vi "HandleObservationSync.vi"(8 "error in (no error)":errorcluster, 11 "S4GUI in":refnum<class "S4GUI.lvclass">) -> (0 "error out":errorcluster, 3 "S4GUI out":refnum<class "S4GUI.lvclass">)   [LabVIEW 2018, in "S4GUI.lvclass"] (continued)
              n490 = Build Array(w1193, w1192, w1191, w1190) -> (w1195:bool[])
              n491 = Boolean Array To Number(Boolean array=w1195) -> (number=w1194:u32)
              n492 = Number To Decimal String(number=w1194) -> (decimal integer string=w1188:string)  [unwired: 1 in]
              n493 = Concatenate Strings("CHANNEL ERROR < " ("string"), w1188, ">: Initialization failed. S4GUI:HandleObservationSync.vi state 252." ("Error Msg")) -> (w1187:string)
              n494 = Bundle By Name(cluster=w1198, "Obs_state"=u32 1, "Error Msg"=w1187) -> (w1197:refnum<class "S4GUI.lvclass">)
            }
            frame 2 {
              n495 = Build Array(w1208, w1207, w1206, w1205) -> (w1204:bool[])
              n496 = Boolean Array To Number(Boolean array=w1204) -> (number=w1200:u32)
              n497 = Number To Decimal String(number=w1200) -> (decimal integer string=w1199:string)  [unwired: 1 in]
              n498 = Concatenate Strings("CHANNEL ERROR < " ("string"), w1199, ">:  Invalid Exposition Time. S4GUI:HandleObservationSync.vi state 252." ("Error Msg")) -> (w1202:string)
              n499 = Bundle By Name(cluster=w1211, "Obs_state"=u32 1, "Error Msg"=w1202) -> (w1210:refnum<class "S4GUI.lvclass">)
            }
            frame 3 {
              n500 = Bundle By Name(cluster=w1215, "Obs_state"=u32 1, "Error Msg"="ERROR: Invalid configuration in the channels. S4GUI:HandleObservationSync.vi state 252.") -> (w1214:refnum<class "S4GUI.lvclass">)
            }
          }
        }
        frame 253 {
          # "Sem SyncBox, \ntrigger mode = 0 (internal)\nCom SyncBox\ntrigger mode = 6 (ext. start)"
          n501 = call-dynamic "Read Sync Box.lvclass.vi"("error in (no error)"=w1327, "SPARC4_AC in"=w1326) -> ("error out"=w1329:errorcluster, "Sync Box.lvclass"=w1330:refnum<class "Sync Box.lvclass">, "SPARC4_AC out"=w1325:refnum<class "S4GUI.lvclass">)  [unwired: 7 in]
          n502 = call "Read connection.vi"("error in (no error)"=w1329, "Server in"=w1330) -> ("error out"=w1328:errorcluster, "connection"=w1290:bool)  [unwired: 7 in, 1 out]
          n503 = case shown="True" w1290 {
            tunnel: [u8 6 ("TRIGGER_MODE") u8 0 ("TRIGGER_MODE")] -> w1307
            frame True {
            }
            frame False {
            }
          }
          n504 = call-dynamic "Read AcquisitionA.vi"("error in (no error)"=w1328, "S4ACS_GUI in"=w1325) -> ("error out"=w1312:errorcluster, "Acquisition.lvclass"=w1313:refnum<class "Acquisition.lvclass">, "S4ACS_GUI out"=w1311:refnum<class "S4GUI.lvclass">)  [unwired: 7 in]
          n505 = call-dynamic "Read Channel.vi"("error in (no error)"=w1312, "Acquisition in"=w1313) -> ("error out"=w1295:errorcluster, "Channel.lvclass"=w1294:refnum<class "Channel.lvclass">, "Acquisition out"=w1322:refnum<class "Acquisition.lvclass">)  [unwired: 7 in]
          n506 = call-dynamic "Read Interface.vi"("error in (no error)"=w1295, "Channel in"=w1294) -> ("error out"=w1293:errorcluster, "Interface.lvclass"=w1299:refnum<class "Interface.lvclass">, "Channel out"=w1298:refnum<class "Channel.lvclass">)  [unwired: 7 in]
          n507 = call-dynamic "Get CCD_Config.vi"("error in (no error)"=w1293, "Interface in"=w1299) -> ("error out"=w1306:errorcluster, "output cluster"=w1308:T1, "Interface out"=w1305:refnum<class "Interface.lvclass">)  [unwired: 7 in]
          n508 = Bundle By Name(cluster=w1308, "TRIGGER_MODE"=w1307) -> (w1304:T1)
          n509 = call-dynamic "Set CCD_Config.vi"("error in (no error)"=w1306, "input cluster"=w1304, "Interface in"=w1305) -> ("error out"=w1302:errorcluster, "Interface out"=w1300:refnum<class "Interface.lvclass">)  [unwired: 7 in]
          n510 = Flatten To String(anything=w1304, error in (no error)=w1302) -> (data string=w1303:string, error out=w1301:errorcluster)  [unwired: 2 in, 1 out]
          n511 = call "Write flatted cluster.vi"("error in (no error)"=w1301, "flatted cluster"=w1303, "Interface in"=w1300) -> ("error out"=w1296:errorcluster, "Interface out"=w1297:refnum<class "Interface.lvclass">)  [unwired: 7 in]
          n512 = Increment(x=w1333) -> (x+1=w1332:u32)
          n513 = call-dynamic "Write Interface.vi"("error in (no error)"=w1296, "Interface.lvclass"=w1297, "Channel in"=w1298) -> ("error out"=w1292:errorcluster, "Channel out"=w1291:refnum<class "Channel.lvclass">)  [unwired: 7 in]
          n514 = call-dynamic "Read State Machine.vi"("error in (no error)"=w1292, "Device in"=w1291) -> ("error out"=w1319:errorcluster, "State Machine.lvclass"=w1321:refnum<class "State Machine.lvclass">, "Device out"=w1317:refnum<class "Channel.lvclass">)  [unwired: 7 in]
          n515 = call "Next State.vi"("error in (no error)"=w1319, "New_State"=60, "State Machine in"=w1321) -> ("error out"=w1314:errorcluster, "State Machine out"=w1315:refnum<class "State Machine.lvclass">)  [unwired: 7 in]
          n516 = call-dynamic "Write State Machine.vi"("error in (no error)"=w1314, "State Machine.lvclass"=w1315, "Device in"=w1317) -> ("error out"=w1316:errorcluster, "Device out"=w1318:refnum<class "Channel.lvclass">)  [unwired: 7 in]
          n517 = call-dynamic "Write Channel.vi"("error in (no error)"=w1316, "Channel.lvclass"=w1318, "Acquisition in"=w1322) -> ("error out"=w1309:errorcluster, "Acquisition out"=w1310:refnum<class "Acquisition.lvclass">)  [unwired: 7 in]
          n518 = call-dynamic "Write AcquisitionA.vi"("error in (no error)"=w1309, "Acquisition.lvclass"=w1310, "S4ACS_GUI in"=w1311) -> ("error out"=w1324:errorcluster, "S4ACS_GUI out"=w1323:refnum<class "S4GUI.lvclass">)  [unwired: 7 in]
          n519 = Bundle By Name(cluster=w1323, "Obs_state"=w1332) -> (w1331:refnum<class "S4GUI.lvclass">)
        }
        frame 254 {
          # "Espera terminar a execução do comando atual \nantes de ir ao proximo passo da Observação."
          n520 = call-dynamic "Read AcquisitionA.vi"("error in (no error)"=w1353, "S4ACS_GUI in"=w1354) -> ("error out"=w1359:errorcluster, "Acquisition.lvclass"=w1360:refnum<class "Acquisition.lvclass">, "S4ACS_GUI out"=w1356:refnum<class "S4GUI.lvclass">)  [unwired: 7 in]
          n521 = call-dynamic "Read Channel.vi"("error in (no error)"=w1359, "Acquisition in"=w1360) -> ("error out"=w1351:errorcluster, "Channel.lvclass"=w1350:refnum<class "Channel.lvclass">, "Acquisition out"=w1358:refnum<class "Acquisition.lvclass">)  [unwired: 7 in]
          n522 = call-dynamic "Read State Machine.vi"("error in (no error)"=w1351, "Device in"=w1350) -> ("error out"=w1342:errorcluster, "State Machine.lvclass"=w1344:refnum<class "State Machine.lvclass">, "Device out"=w1348:refnum<class "Channel.lvclass">)  [unwired: 7 in]
          n523 = call-dynamic "Read State.vi"("error in (no error)"=w1342, "State Machine in"=w1344) -> ("error out"=w1341:errorcluster, "State"=w1338:i32, "State Machine out"=w1343:refnum<class "State Machine.lvclass">)  [unwired: 7 in]
          n524 = Equal To 0?(x=w1338) -> (x = 0?=w1340:bool)
          n525 = call-dynamic "Write State Machine.vi"("error in (no error)"=w1341, "State Machine.lvclass"=w1343, "Device in"=w1348) -> ("error out"=w1347:errorcluster, "Device out"=w1349:refnum<class "Channel.lvclass">)  [unwired: 7 in]
          n526 = call-dynamic "Write Channel.vi"("error in (no error)"=w1347, "Channel.lvclass"=w1349, "Acquisition in"=w1358) -> ("error out"=w1355:errorcluster, "Acquisition out"=w1357:refnum<class "Acquisition.lvclass">)  [unwired: 7 in]
          n527 = disable-structure shown="Enabled" {
            disable-tunnel: [u32 299 ("t") w1362] -> w1337
            disable-tunnel: w1336 -> [_ w1363]
            frame Disabled {
            }
            frame Enabled {
              n528 = Increment(x=w1363) -> (x+1=w1362:u32)
            }
          }
          n529 = Select(t=w1337, s=w1340, f=w1336) -> (s? t:f=w1339:u32)
          n530 = call-dynamic "Write AcquisitionA.vi"("error in (no error)"=w1355, "Acquisition.lvclass"=w1357, "S4ACS_GUI in"=w1356) -> ("error out"=w1352:errorcluster, "S4ACS_GUI out"=w1346:refnum<class "S4GUI.lvclass">)  [unwired: 7 in]
          n531 = Bundle By Name(cluster=w1346, "Obs_state"=w1339) -> (w1345:refnum<class "S4GUI.lvclass">)
        }
        frame 255 {
          n532 = call "Read AcquisitionB.vi"("error in (no error)"=w1374, "S4ACS_GUI in"=w1375) -> ("error out"=w1367:errorcluster, "Acquisition.lvclass"=w1368:refnum<class "Acquisition.lvclass">, "S4ACS_GUI out"=w1377:refnum<class "S4GUI.lvclass">)  [unwired: 7 in]
          n533 = call "Read connection.vi"("error in (no error)"=w1367, "Server in"=w1368) -> ("error out"=w1366:errorcluster, "connection"=w1364:bool, "Server out"=w1365:refnum<class "Acquisition.lvclass">)  [unwired: 7 in]
          n534 = case shown="False" w1364 {
            tunnel: w1365 -> [w1385 w1405]
            tunnel: w1366 -> [w1384 w1404]
            tunnel: [w1385 w1402] -> w1378
            tunnel: [w1384 w1401] -> w1376
            tunnel: w1371 -> [w1383 w1394]
            tunnel: [w1379 w1393] -> w1370
            frame False {
              n535 = Increment(x=w1383) -> (x+1=w1382:u32)
              n536 = Increment(x=w1382) -> (x+1=w1381:u32)
              n537 = Increment(x=w1381) -> (x+1=w1380:u32)
              n538 = Increment(x=w1380) -> (x+1=w1379:u32)
            }
            frame True {
              # "configura o canal,\nmas não dispara\na exposicao."
              n539 = call-dynamic "Read Channel.vi"("error in (no error)"=w1404, "Acquisition in"=w1405) -> ("error out"=w1390:errorcluster, "Channel.lvclass"=w1392:refnum<class "Channel.lvclass">, "Acquisition out"=w1403:refnum<class "Acquisition.lvclass">)  [unwired: 7 in]
              n540 = call-dynamic "Write expose.vi"("error in (no error)"=w1390, "expose"=FALSE, "Channel in"=w1392) -> ("error out"=w1389:errorcluster, "Channel out"=w1391:refnum<class "Channel.lvclass">)  [unwired: 7 in]
              n541 = call-dynamic "Read State Machine.vi"("error in (no error)"=w1389, "Device in"=w1391) -> ("error out"=w1398:errorcluster, "State Machine.lvclass"=w1400:refnum<class "State Machine.lvclass">, "Device out"=w1396:refnum<class "Channel.lvclass">)  [unwired: 7 in]
              n542 = call "Next State.vi"("error in (no error)"=w1398, "New_State"=1, "State Machine in"=w1400) -> ("error out"=w1386:errorcluster, "State Machine out"=w1387:refnum<class "State Machine.lvclass">)  [unwired: 7 in]
              n543 = Increment(x=w1394) -> (x+1=w1393:u32)
              n544 = call-dynamic "Write State Machine.vi"("error in (no error)"=w1386, "State Machine.lvclass"=w1387, "Device in"=w1396) -> ("error out"=w1395:errorcluster, "Device out"=w1397:refnum<class "Channel.lvclass">)  [unwired: 7 in]
              n545 = call-dynamic "Write Channel.vi"("error in (no error)"=w1395, "Channel.lvclass"=w1397, "Acquisition in"=w1403) -> ("error out"=w1401:errorcluster, "Acquisition out"=w1402:refnum<class "Acquisition.lvclass">)  [unwired: 7 in]
            }
          }
          n546 = call "Write AcquisitionB.vi"("error in (no error)"=w1376, "Acquisition.lvclass"=w1378, "S4ACS_GUI in"=w1377) -> ("error out"=w1373:errorcluster, "S4ACS_GUI out"=w1372:refnum<class "S4GUI.lvclass">)  [unwired: 7 in]
          n547 = Bundle By Name(cluster=w1372, "Obs_state"=w1370) -> (w1369:refnum<class "S4GUI.lvclass">)
        }
        frame 256 {
          # "Espera terminar a execução do comando atual \nantes de ir ao proximo passo da Observação."
          n548 = call "Read AcquisitionB.vi"("error in (no error)"=w1423, "S4ACS_GUI in"=w1424) -> ("error out"=w1429:errorcluster, "Acquisition.lvclass"=w1430:refnum<class "Acquisition.lvclass">, "S4ACS_GUI out"=w1426:refnum<class "S4GUI.lvclass">)  [unwired: 7 in]
          n549 = call-dynamic "Read Channel.vi"("error in (no error)"=w1429, "Acquisition in"=w1430) -> ("error out"=w1421:errorcluster, "Channel.lvclass"=w1420:refnum<class "Channel.lvclass">, "Acquisition out"=w1428:refnum<class "Acquisition.lvclass">)  [unwired: 7 in]
          n550 = call-dynamic "Read State Machine.vi"("error in (no error)"=w1421, "Device in"=w1420) -> ("error out"=w1412:errorcluster, "State Machine.lvclass"=w1414:refnum<class "State Machine.lvclass">, "Device out"=w1418:refnum<class "Channel.lvclass">)  [unwired: 7 in]
          n551 = call-dynamic "Read State.vi"("error in (no error)"=w1412, "State Machine in"=w1414) -> ("error out"=w1411:errorcluster, "State"=w1408:i32, "State Machine out"=w1413:refnum<class "State Machine.lvclass">)  [unwired: 7 in]
          n552 = call-dynamic "Write State Machine.vi"("error in (no error)"=w1411, "State Machine.lvclass"=w1413, "Device in"=w1418) -> ("error out"=w1417:errorcluster, "Device out"=w1419:refnum<class "Channel.lvclass">)  [unwired: 7 in]
          n553 = call-dynamic "Write Channel.vi"("error in (no error)"=w1417, "Channel.lvclass"=w1419, "Acquisition in"=w1428) -> ("error out"=w1425:errorcluster, "Acquisition out"=w1427:refnum<class "Acquisition.lvclass">)  [unwired: 7 in]
          n554 = Equal To 0?(x=w1408) -> (x = 0?=w1410:bool)
          n555 = disable-structure shown="Enabled" {
            disable-tunnel: [u32 299 ("t") w1432] -> w1406
            disable-tunnel: w1407 -> [_ w1435]
            frame Disabled {
            }
            frame Enabled {
              n556 = Increment(x=w1435) -> (x+1=w1434:u32)
              n557 = Increment(x=w1434) -> (x+1=w1433:u32)
              n558 = Increment(x=w1433) -> (x+1=w1432:u32)
            }
          }
          n559 = Select(t=w1406, s=w1410, f=w1407) -> (s? t:f=w1409:u32)
          n560 = call "Write AcquisitionB.vi"("error in (no error)"=w1425, "Acquisition.lvclass"=w1427, "S4ACS_GUI in"=w1426) -> ("error out"=w1422:errorcluster, "S4ACS_GUI out"=w1416:refnum<class "S4GUI.lvclass">)  [unwired: 7 in]
          n561 = Bundle By Name(cluster=w1416, "Obs_state"=w1409) -> (w1415:refnum<class "S4GUI.lvclass">)
        }
        frame 257 {
          # "Sem SyncBox, \ntrigger mode = 0 (internal)\nCom SyncBox\ntrigger mode = 6 (ext. start)"
          n562 = call-dynamic "Read Sync Box.lvclass.vi"("error in (no error)"=w1473, "SPARC4_AC in"=w1472) -> ("error out"=w1475:errorcluster, "Sync Box.lvclass"=w1476:refnum<class "Sync Box.lvclass">, "SPARC4_AC out"=w1471:refnum<class "S4GUI.lvclass">)  [unwired: 7 in]
          n563 = call "Read connection.vi"("error in (no error)"=w1475, "Server in"=w1476) -> ("error out"=w1474:errorcluster, "connection"=w1437:bool)  [unwired: 7 in, 1 out]
          n564 = case shown="False" w1437 {
            tunnel: [u8 6 ("TRIGGER_MODE") u8 0 ("TRIGGER_MODE")] -> w1436
            frame True {
            }
            frame False {
            }
          }
          n565 = call "Read AcquisitionB.vi"("error in (no error)"=w1474, "S4ACS_GUI in"=w1471) -> ("error out"=w1458:errorcluster, "Acquisition.lvclass"=w1459:refnum<class "Acquisition.lvclass">, "S4ACS_GUI out"=w1457:refnum<class "S4GUI.lvclass">)  [unwired: 7 in]
          n566 = call-dynamic "Read Channel.vi"("error in (no error)"=w1458, "Acquisition in"=w1459) -> ("error out"=w1442:errorcluster, "Channel.lvclass"=w1441:refnum<class "Channel.lvclass">, "Acquisition out"=w1468:refnum<class "Acquisition.lvclass">)  [unwired: 7 in]
          n567 = call-dynamic "Read Interface.vi"("error in (no error)"=w1442, "Channel in"=w1441) -> ("error out"=w1440:errorcluster, "Interface.lvclass"=w1446:refnum<class "Interface.lvclass">, "Channel out"=w1445:refnum<class "Channel.lvclass">)  [unwired: 7 in]
          n568 = call-dynamic "Get CCD_Config.vi"("error in (no error)"=w1440, "Interface in"=w1446) -> ("error out"=w1453:errorcluster, "output cluster"=w1454:T1, "Interface out"=w1452:refnum<class "Interface.lvclass">)  [unwired: 7 in]
          n569 = Bundle By Name(cluster=w1454, "TRIGGER_MODE"=w1436) -> (w1451:T1)
          n570 = call-dynamic "Set CCD_Config.vi"("error in (no error)"=w1453, "input cluster"=w1451, "Interface in"=w1452) -> ("error out"=w1449:errorcluster, "Interface out"=w1447:refnum<class "Interface.lvclass">)  [unwired: 7 in]
          n571 = Flatten To String(anything=w1451, error in (no error)=w1449) -> (data string=w1450:string, error out=w1448:errorcluster)  [unwired: 2 in, 1 out]
          n572 = call "Write flatted cluster.vi"("error in (no error)"=w1448, "flatted cluster"=w1450, "Interface in"=w1447) -> ("error out"=w1443:errorcluster, "Interface out"=w1444:refnum<class "Interface.lvclass">)  [unwired: 7 in]
          n573 = Increment(x=w1479) -> (x+1=w1478:u32)
          n574 = call-dynamic "Write Interface.vi"("error in (no error)"=w1443, "Interface.lvclass"=w1444, "Channel in"=w1445) -> ("error out"=w1439:errorcluster, "Channel out"=w1438:refnum<class "Channel.lvclass">)  [unwired: 7 in]
          n575 = call-dynamic "Read State Machine.vi"("error in (no error)"=w1439, "Device in"=w1438) -> ("error out"=w1465:errorcluster, "State Machine.lvclass"=w1467:refnum<class "State Machine.lvclass">, "Device out"=w1463:refnum<class "Channel.lvclass">)  [unwired: 7 in]
          n576 = call "Next State.vi"("error in (no error)"=w1465, "New_State"=60, "State Machine in"=w1467) -> ("error out"=w1460:errorcluster, "State Machine out"=w1461:refnum<class "State Machine.lvclass">)  [unwired: 7 in]
          n577 = call-dynamic "Write State Machine.vi"("error in (no error)"=w1460, "State Machine.lvclass"=w1461, "Device in"=w1463) -> ("error out"=w1462:errorcluster, "Device out"=w1464:refnum<class "Channel.lvclass">)  [unwired: 7 in]
          n578 = call-dynamic "Write Channel.vi"("error in (no error)"=w1462, "Channel.lvclass"=w1464, "Acquisition in"=w1468) -> ("error out"=w1455:errorcluster, "Acquisition out"=w1456:refnum<class "Acquisition.lvclass">)  [unwired: 7 in]
          n579 = call "Write AcquisitionB.vi"("error in (no error)"=w1455, "Acquisition.lvclass"=w1456, "S4ACS_GUI in"=w1457) -> ("error out"=w1470:errorcluster, "S4ACS_GUI out"=w1469:refnum<class "S4GUI.lvclass">)  [unwired: 7 in]
          n580 = Bundle By Name(cluster=w1469, "Obs_state"=w1478) -> (w1477:refnum<class "S4GUI.lvclass">)
        }
        frame 258 {
          # "Espera terminar a execução do comando atual \nantes de ir ao proximo passo da Observação."
          n581 = call "Read AcquisitionB.vi"("error in (no error)"=w1499, "S4ACS_GUI in"=w1500) -> ("error out"=w1505:errorcluster, "Acquisition.lvclass"=w1506:refnum<class "Acquisition.lvclass">, "S4ACS_GUI out"=w1502:refnum<class "S4GUI.lvclass">)  [unwired: 7 in]
          n582 = call-dynamic "Read Channel.vi"("error in (no error)"=w1505, "Acquisition in"=w1506) -> ("error out"=w1497:errorcluster, "Channel.lvclass"=w1496:refnum<class "Channel.lvclass">, "Acquisition out"=w1504:refnum<class "Acquisition.lvclass">)  [unwired: 7 in]
          n583 = call-dynamic "Read State Machine.vi"("error in (no error)"=w1497, "Device in"=w1496) -> ("error out"=w1488:errorcluster, "State Machine.lvclass"=w1490:refnum<class "State Machine.lvclass">, "Device out"=w1494:refnum<class "Channel.lvclass">)  [unwired: 7 in]
          n584 = call-dynamic "Read State.vi"("error in (no error)"=w1488, "State Machine in"=w1490) -> ("error out"=w1487:errorcluster, "State"=w1484:i32, "State Machine out"=w1489:refnum<class "State Machine.lvclass">)  [unwired: 7 in]
          n585 = call-dynamic "Write State Machine.vi"("error in (no error)"=w1487, "State Machine.lvclass"=w1489, "Device in"=w1494) -> ("error out"=w1493:errorcluster, "Device out"=w1495:refnum<class "Channel.lvclass">)  [unwired: 7 in]
          n586 = call-dynamic "Write Channel.vi"("error in (no error)"=w1493, "Channel.lvclass"=w1495, "Acquisition in"=w1504) -> ("error out"=w1501:errorcluster, "Acquisition out"=w1503:refnum<class "Acquisition.lvclass">)  [unwired: 7 in]
          n587 = Equal To 0?(x=w1484) -> (x = 0?=w1486:bool)
          n588 = Increment(x=w1483) -> (x+1=w1482:u32)
          n589 = Select(t=w1482, s=w1486, f=w1483) -> (s? t:f=w1485:u32)
          n590 = call "Write AcquisitionB.vi"("error in (no error)"=w1501, "Acquisition.lvclass"=w1503, "S4ACS_GUI in"=w1502) -> ("error out"=w1498:errorcluster, "S4ACS_GUI out"=w1492:refnum<class "S4GUI.lvclass">)  [unwired: 7 in]
          n591 = Bundle By Name(cluster=w1492, "Obs_state"=w1485) -> (w1491:refnum<class "S4GUI.lvclass">)
        }
        frame 259 {
          n592 = call-dynamic "Read AcquisitionC.vi"("error in (no error)"=w1517, "S4ACS_GUI in"=w1518) -> ("error out"=w1509:errorcluster, "Acquisition.lvclass"=w1511:refnum<class "Acquisition.lvclass">, "S4ACS_GUI out"=w1520:refnum<class "S4GUI.lvclass">)  [unwired: 7 in]
          n593 = call "Read connection.vi"("error in (no error)"=w1509, "Server in"=w1511) -> ("error out"=w1508:errorcluster, "connection"=w1507:bool, "Server out"=w1510:refnum<class "Acquisition.lvclass">)  [unwired: 7 in]
          n594 = case shown="True" w1507 {
            tunnel: w1510 -> [w1527 w1548]
            tunnel: w1508 -> [w1528 w1547]
            tunnel: [w1527 w1545] -> w1521
            tunnel: [w1528 w1544] -> w1519
            tunnel: w1514 -> [w1526 w1537]
            tunnel: [w1522 w1536] -> w1513
            frame False {
              n595 = Increment(x=w1526) -> (x+1=w1525:u32)
              n596 = Increment(x=w1525) -> (x+1=w1524:u32)
              n597 = Increment(x=w1524) -> (x+1=w1523:u32)
              n598 = Increment(x=w1523) -> (x+1=w1522:u32)
            }
            frame True {
              # "configura o canal,\nmas não dispara\na exposicao."
              n599 = call-dynamic "Read Channel.vi"("error in (no error)"=w1547, "Acquisition in"=w1548) -> ("error out"=w1533:errorcluster, "Channel.lvclass"=w1535:refnum<class "Channel.lvclass">, "Acquisition out"=w1546:refnum<class "Acquisition.lvclass">)  [unwired: 7 in]
              n600 = call-dynamic "Write expose.vi"("error in (no error)"=w1533, "expose"=FALSE, "Channel in"=w1535) -> ("error out"=w1532:errorcluster, "Channel out"=w1534:refnum<class "Channel.lvclass">)  [unwired: 7 in]
              n601 = call-dynamic "Read State Machine.vi"("error in (no error)"=w1532, "Device in"=w1534) -> ("error out"=w1541:errorcluster, "State Machine.lvclass"=w1543:refnum<class "State Machine.lvclass">, "Device out"=w1539:refnum<class "Channel.lvclass">)  [unwired: 7 in]
              n602 = call "Next State.vi"("error in (no error)"=w1541, "New_State"=1, "State Machine in"=w1543) -> ("error out"=w1529:errorcluster, "State Machine out"=w1530:refnum<class "State Machine.lvclass">)  [unwired: 7 in]
              n603 = Increment(x=w1537) -> (x+1=w1536:u32)
              n604 = call-dynamic "Write State Machine.vi"("error in (no error)"=w1529, "State Machine.lvclass"=w1530, "Device in"=w1539) -> ("error out"=w1538:errorcluster, "Device out"=w1540:refnum<class "Channel.lvclass">)  [unwired: 7 in]
              n605 = call-dynamic "Write Channel.vi"("error in (no error)"=w1538, "Channel.lvclass"=w1540, "Acquisition in"=w1546) -> ("error out"=w1544:errorcluster, "Acquisition out"=w1545:refnum<class "Acquisition.lvclass">)  [unwired: 7 in]
            }
          }
          n606 = call-dynamic "Write AcquisitionC.vi"("error in (no error)"=w1519, "Acquisition.lvclass"=w1521, "S4ACS_GUI in"=w1520) -> ("error out"=w1516:errorcluster, "S4ACS_GUI out"=w1515:refnum<class "S4GUI.lvclass">)  [unwired: 7 in]
          n607 = Bundle By Name(cluster=w1515, "Obs_state"=w1513) -> (w1512:refnum<class "S4GUI.lvclass">)
        }
        frame 260 {
          # "Espera terminar a execução do comando atual \nantes de ir ao proximo passo da Observação."
          n608 = call-dynamic "Read AcquisitionC.vi"("error in (no error)"=w1566, "S4ACS_GUI in"=w1567) -> ("error out"=w1572:errorcluster, "Acquisition.lvclass"=w1573:refnum<class "Acquisition.lvclass">, "S4ACS_GUI out"=w1569:refnum<class "S4GUI.lvclass">)  [unwired: 7 in]
          n609 = call-dynamic "Read Channel.vi"("error in (no error)"=w1572, "Acquisition in"=w1573) -> ("error out"=w1564:errorcluster, "Channel.lvclass"=w1563:refnum<class "Channel.lvclass">, "Acquisition out"=w1571:refnum<class "Acquisition.lvclass">)  [unwired: 7 in]
          n610 = call-dynamic "Read State Machine.vi"("error in (no error)"=w1564, "Device in"=w1563) -> ("error out"=w1555:errorcluster, "State Machine.lvclass"=w1557:refnum<class "State Machine.lvclass">, "Device out"=w1561:refnum<class "Channel.lvclass">)  [unwired: 7 in]
          n611 = call-dynamic "Read State.vi"("error in (no error)"=w1555, "State Machine in"=w1557) -> ("error out"=w1554:errorcluster, "State"=w1551:i32, "State Machine out"=w1556:refnum<class "State Machine.lvclass">)  [unwired: 7 in]
          n612 = Equal To 0?(x=w1551) -> (x = 0?=w1553:bool)
          n613 = call-dynamic "Write State Machine.vi"("error in (no error)"=w1554, "State Machine.lvclass"=w1556, "Device in"=w1561) -> ("error out"=w1560:errorcluster, "Device out"=w1562:refnum<class "Channel.lvclass">)  [unwired: 7 in]
          n614 = call-dynamic "Write Channel.vi"("error in (no error)"=w1560, "Channel.lvclass"=w1562, "Acquisition in"=w1571) -> ("error out"=w1568:errorcluster, "Acquisition out"=w1570:refnum<class "Acquisition.lvclass">)  [unwired: 7 in]
          n615 = disable-structure shown="Enabled" {
            disable-tunnel: [u32 299 ("t") w1575] -> w1549
            disable-tunnel: w1550 -> [_ w1578]
            frame Disabled {
            }
            frame Enabled {
              n616 = Increment(x=w1578) -> (x+1=w1577:u32)
              n617 = Increment(x=w1577) -> (x+1=w1576:u32)
              n618 = Increment(x=w1576) -> (x+1=w1575:u32)
            }
          }
          n619 = Select(t=w1549, s=w1553, f=w1550) -> (s? t:f=w1552:u32)
          n620 = call-dynamic "Write AcquisitionC.vi"("error in (no error)"=w1568, "Acquisition.lvclass"=w1570, "S4ACS_GUI in"=w1569) -> ("error out"=w1565:errorcluster, "S4ACS_GUI out"=w1559:refnum<class "S4GUI.lvclass">)  [unwired: 7 in]
          n621 = Bundle By Name(cluster=w1559, "Obs_state"=w1552) -> (w1558:refnum<class "S4GUI.lvclass">)
        }
        frame 261 {
          # "Sem SyncBox, \ntrigger mode = 0 (internal)\nCom SyncBox\ntrigger mode = 6 (ext. start)"
          n622 = call-dynamic "Read Sync Box.lvclass.vi"("error in (no error)"=w1616, "SPARC4_AC in"=w1615) -> ("error out"=w1618:errorcluster, "Sync Box.lvclass"=w1619:refnum<class "Sync Box.lvclass">, "SPARC4_AC out"=w1614:refnum<class "S4GUI.lvclass">)  [unwired: 7 in]
          n623 = call "Read connection.vi"("error in (no error)"=w1618, "Server in"=w1619) -> ("error out"=w1617:errorcluster, "connection"=w1580:bool)  [unwired: 7 in, 1 out]
          n624 = case shown="False" w1580 {
            tunnel: [u8 6 ("TRIGGER_MODE") u8 0 ("TRIGGER_MODE")] -> w1579
            frame True {
            }
            frame False {
            }
          }
          n625 = call-dynamic "Read AcquisitionC.vi"("error in (no error)"=w1617, "S4ACS_GUI in"=w1614) -> ("error out"=w1601:errorcluster, "Acquisition.lvclass"=w1602:refnum<class "Acquisition.lvclass">, "S4ACS_GUI out"=w1600:refnum<class "S4GUI.lvclass">)  [unwired: 7 in]
          n626 = call-dynamic "Read Channel.vi"("error in (no error)"=w1601, "Acquisition in"=w1602) -> ("error out"=w1585:errorcluster, "Channel.lvclass"=w1584:refnum<class "Channel.lvclass">, "Acquisition out"=w1611:refnum<class "Acquisition.lvclass">)  [unwired: 7 in]
          n627 = call-dynamic "Read Interface.vi"("error in (no error)"=w1585, "Channel in"=w1584) -> ("error out"=w1583:errorcluster, "Interface.lvclass"=w1589:refnum<class "Interface.lvclass">, "Channel out"=w1588:refnum<class "Channel.lvclass">)  [unwired: 7 in]
          n628 = call-dynamic "Get CCD_Config.vi"("error in (no error)"=w1583, "Interface in"=w1589) -> ("error out"=w1596:errorcluster, "output cluster"=w1597:T1, "Interface out"=w1595:refnum<class "Interface.lvclass">)  [unwired: 7 in]
          n629 = Bundle By Name(cluster=w1597, "TRIGGER_MODE"=w1579) -> (w1594:T1)
          n630 = call-dynamic "Set CCD_Config.vi"("error in (no error)"=w1596, "input cluster"=w1594, "Interface in"=w1595) -> ("error out"=w1592:errorcluster, "Interface out"=w1590:refnum<class "Interface.lvclass">)  [unwired: 7 in]
          n631 = Flatten To String(anything=w1594, error in (no error)=w1592) -> (data string=w1593:string, error out=w1591:errorcluster)  [unwired: 2 in, 1 out]
          n632 = call "Write flatted cluster.vi"("error in (no error)"=w1591, "flatted cluster"=w1593, "Interface in"=w1590) -> ("error out"=w1586:errorcluster, "Interface out"=w1587:refnum<class "Interface.lvclass">)  [unwired: 7 in]
          n633 = Increment(x=w1622) -> (x+1=w1621:u32)
          n634 = call-dynamic "Write Interface.vi"("error in (no error)"=w1586, "Interface.lvclass"=w1587, "Channel in"=w1588) -> ("error out"=w1582:errorcluster, "Channel out"=w1581:refnum<class "Channel.lvclass">)  [unwired: 7 in]
          n635 = call-dynamic "Read State Machine.vi"("error in (no error)"=w1582, "Device in"=w1581) -> ("error out"=w1608:errorcluster, "State Machine.lvclass"=w1610:refnum<class "State Machine.lvclass">, "Device out"=w1606:refnum<class "Channel.lvclass">)  [unwired: 7 in]
          n636 = call "Next State.vi"("error in (no error)"=w1608, "New_State"=60, "State Machine in"=w1610) -> ("error out"=w1603:errorcluster, "State Machine out"=w1604:refnum<class "State Machine.lvclass">)  [unwired: 7 in]
          n637 = call-dynamic "Write State Machine.vi"("error in (no error)"=w1603, "State Machine.lvclass"=w1604, "Device in"=w1606) -> ("error out"=w1605:errorcluster, "Device out"=w1607:refnum<class "Channel.lvclass">)  [unwired: 7 in]
          n638 = call-dynamic "Write Channel.vi"("error in (no error)"=w1605, "Channel.lvclass"=w1607, "Acquisition in"=w1611) -> ("error out"=w1598:errorcluster, "Acquisition out"=w1599:refnum<class "Acquisition.lvclass">)  [unwired: 7 in]
          n639 = call-dynamic "Write AcquisitionC.vi"("error in (no error)"=w1598, "Acquisition.lvclass"=w1599, "S4ACS_GUI in"=w1600) -> ("error out"=w1613:errorcluster, "S4ACS_GUI out"=w1612:refnum<class "S4GUI.lvclass">)  [unwired: 7 in]
          n640 = Bundle By Name(cluster=w1612, "Obs_state"=w1621) -> (w1620:refnum<class "S4GUI.lvclass">)
        }
        frame 262 {
          # "Espera terminar a execução do comando atual \nantes de ir ao proximo passo da Observação."
          n641 = call-dynamic "Read AcquisitionC.vi"("error in (no error)"=w1642, "S4ACS_GUI in"=w1643) -> ("error out"=w1648:errorcluster, "Acquisition.lvclass"=w1649:refnum<class "Acquisition.lvclass">, "S4ACS_GUI out"=w1645:refnum<class "S4GUI.lvclass">)  [unwired: 7 in]
          n642 = call-dynamic "Read Channel.vi"("error in (no error)"=w1648, "Acquisition in"=w1649) -> ("error out"=w1640:errorcluster, "Channel.lvclass"=w1639:refnum<class "Channel.lvclass">, "Acquisition out"=w1647:refnum<class "Acquisition.lvclass">)  [unwired: 7 in]
          n643 = call-dynamic "Read State Machine.vi"("error in (no error)"=w1640, "Device in"=w1639) -> ("error out"=w1631:errorcluster, "State Machine.lvclass"=w1633:refnum<class "State Machine.lvclass">, "Device out"=w1637:refnum<class "Channel.lvclass">)  [unwired: 7 in]
          n644 = call-dynamic "Read State.vi"("error in (no error)"=w1631, "State Machine in"=w1633) -> ("error out"=w1630:errorcluster, "State"=w1627:i32, "State Machine out"=w1632:refnum<class "State Machine.lvclass">)  [unwired: 7 in]
          n645 = Equal To 0?(x=w1627) -> (x = 0?=w1629:bool)
          n646 = call-dynamic "Write State Machine.vi"("error in (no error)"=w1630, "State Machine.lvclass"=w1632, "Device in"=w1637) -> ("error out"=w1636:errorcluster, "Device out"=w1638:refnum<class "Channel.lvclass">)  [unwired: 7 in]
          n647 = call-dynamic "Write Channel.vi"("error in (no error)"=w1636, "Channel.lvclass"=w1638, "Acquisition in"=w1647) -> ("error out"=w1644:errorcluster, "Acquisition out"=w1646:refnum<class "Acquisition.lvclass">)  [unwired: 7 in]
          n648 = Increment(x=w1626) -> (x+1=w1625:u32)
          n649 = Select(t=w1625, s=w1629, f=w1626) -> (s? t:f=w1628:u32)
          n650 = call-dynamic "Write AcquisitionC.vi"("error in (no error)"=w1644, "Acquisition.lvclass"=w1646, "S4ACS_GUI in"=w1645) -> ("error out"=w1641:errorcluster, "S4ACS_GUI out"=w1635:refnum<class "S4GUI.lvclass">)  [unwired: 7 in]
          n651 = Bundle By Name(cluster=w1635, "Obs_state"=w1628) -> (w1634:refnum<class "S4GUI.lvclass">)
        }
        frame 263 {
          # "Dispara o comando para o dispositivo corrente."
          n652 = call-dynamic "Read AcquisitionD.vi"("error in (no error)"=w1660, "S4ACS_GUI in"=w1661) -> ("error out"=w1653:errorcluster, "Acquisition.lvclass"=w1654:refnum<class "Acquisition.lvclass">, "S4ACS_GUI out"=w1663:refnum<class "S4GUI.lvclass">)  [unwired: 7 in]
          n653 = call "Read connection.vi"("error in (no error)"=w1653, "Server in"=w1654) -> ("error out"=w1651:errorcluster, "connection"=w1650:bool, "Server out"=w1652:refnum<class "Acquisition.lvclass">)  [unwired: 7 in]
          n654 = case shown="True" w1650 {
            tunnel: w1652 -> [w1667 w1687]
            tunnel: w1651 -> [w1666 w1686]
            tunnel: [w1667 w1684] -> w1664
            tunnel: [w1666 w1683] -> w1662
            tunnel: w1657 -> [_ w1676]
            tunnel: [u32 299 w1675] -> w1656
            frame False {
            }
            frame True {
              # "configura o canal,\nmas não dispara\na exposicao."
              n655 = call-dynamic "Read Channel.vi"("error in (no error)"=w1686, "Acquisition in"=w1687) -> ("error out"=w1672:errorcluster, "Channel.lvclass"=w1674:refnum<class "Channel.lvclass">, "Acquisition out"=w1685:refnum<class "Acquisition.lvclass">)  [unwired: 7 in]
              n656 = call-dynamic "Write expose.vi"("error in (no error)"=w1672, "expose"=FALSE, "Channel in"=w1674) -> ("error out"=w1671:errorcluster, "Channel out"=w1673:refnum<class "Channel.lvclass">)  [unwired: 7 in]
              n657 = call-dynamic "Read State Machine.vi"("error in (no error)"=w1671, "Device in"=w1673) -> ("error out"=w1680:errorcluster, "State Machine.lvclass"=w1682:refnum<class "State Machine.lvclass">, "Device out"=w1678:refnum<class "Channel.lvclass">)  [unwired: 7 in]
              n658 = call "Next State.vi"("error in (no error)"=w1680, "New_State"=1, "State Machine in"=w1682) -> ("error out"=w1668:errorcluster, "State Machine out"=w1669:refnum<class "State Machine.lvclass">)  [unwired: 7 in]
              n659 = Increment(x=w1676) -> (x+1=w1675:u32)
              n660 = call-dynamic "Write State Machine.vi"("error in (no error)"=w1668, "State Machine.lvclass"=w1669, "Device in"=w1678) -> ("error out"=w1677:errorcluster, "Device out"=w1679:refnum<class "Channel.lvclass">)  [unwired: 7 in]
              n661 = call-dynamic "Write Channel.vi"("error in (no error)"=w1677, "Channel.lvclass"=w1679, "Acquisition in"=w1685) -> ("error out"=w1683:errorcluster, "Acquisition out"=w1684:refnum<class "Acquisition.lvclass">)  [unwired: 7 in]
            }
          }
          n662 = call-dynamic "Write AcquisitionD.vi"("error in (no error)"=w1662, "Acquisition.lvclass"=w1664, "S4ACS_GUI in"=w1663) -> ("error out"=w1659:errorcluster, "S4ACS_GUI out"=w1658:refnum<class "S4GUI.lvclass">)  [unwired: 7 in]
          n663 = Bundle By Name(cluster=w1658, "Obs_state"=w1656) -> (w1655:refnum<class "S4GUI.lvclass">)
        }
        frame 264 {
          # "Espera terminar a execução do comando atual \nantes de ir ao proximo passo da Observação."
          n664 = call-dynamic "Read AcquisitionD.vi"("error in (no error)"=w1705, "S4ACS_GUI in"=w1706) -> ("error out"=w1711:errorcluster, "Acquisition.lvclass"=w1712:refnum<class "Acquisition.lvclass">, "S4ACS_GUI out"=w1708:refnum<class "S4GUI.lvclass">)  [unwired: 7 in]
          n665 = call-dynamic "Read Channel.vi"("error in (no error)"=w1711, "Acquisition in"=w1712) -> ("error out"=w1703:errorcluster, "Channel.lvclass"=w1702:refnum<class "Channel.lvclass">, "Acquisition out"=w1710:refnum<class "Acquisition.lvclass">)  [unwired: 7 in]
          n666 = call-dynamic "Read State Machine.vi"("error in (no error)"=w1703, "Device in"=w1702) -> ("error out"=w1694:errorcluster, "State Machine.lvclass"=w1696:refnum<class "State Machine.lvclass">, "Device out"=w1700:refnum<class "Channel.lvclass">)  [unwired: 7 in]
          n667 = call-dynamic "Read State.vi"("error in (no error)"=w1694, "State Machine in"=w1696) -> ("error out"=w1693:errorcluster, "State"=w1690:i32, "State Machine out"=w1695:refnum<class "State Machine.lvclass">)  [unwired: 7 in]
          n668 = Equal To 0?(x=w1690) -> (x = 0?=w1692:bool)
          n669 = call-dynamic "Write State Machine.vi"("error in (no error)"=w1693, "State Machine.lvclass"=w1695, "Device in"=w1700) -> ("error out"=w1699:errorcluster, "Device out"=w1701:refnum<class "Channel.lvclass">)  [unwired: 7 in]
          n670 = call-dynamic "Write Channel.vi"("error in (no error)"=w1699, "Channel.lvclass"=w1701, "Acquisition in"=w1710) -> ("error out"=w1707:errorcluster, "Acquisition out"=w1709:refnum<class "Acquisition.lvclass">)  [unwired: 7 in]
          n671 = disable-structure shown="Enabled" {
            disable-tunnel: w1689 -> [w1714 _]
            disable-tunnel: [w1713 u32 299] -> w1688
            frame Disabled {
              n672 = Increment(x=w1714) -> (x+1=w1713:u32)
            }
            frame Enabled {
            }
          }
          n673 = Select(t=w1688, s=w1692, f=w1689) -> (s? t:f=w1691:u32)
          n674 = call-dynamic "Write AcquisitionD.vi"("error in (no error)"=w1707, "Acquisition.lvclass"=w1709, "S4ACS_GUI in"=w1708) -> ("error out"=w1704:errorcluster, "S4ACS_GUI out"=w1698:refnum<class "S4GUI.lvclass">)  [unwired: 7 in]
          n675 = Bundle By Name(cluster=w1698, "Obs_state"=w1691) -> (w1697:refnum<class "S4GUI.lvclass">)
        }
        frame 265 {
          # "Sem SyncBox, \ntrigger mode = 0 (internal)\nCom SyncBox\ntrigger mode = 6 (ext. start)"
          n676 = call-dynamic "Read Sync Box.lvclass.vi"("error in (no error)"=w1753, "SPARC4_AC in"=w1752) -> ("error out"=w1755:errorcluster, "Sync Box.lvclass"=w1756:refnum<class "Sync Box.lvclass">, "SPARC4_AC out"=w1751:refnum<class "S4GUI.lvclass">)  [unwired: 7 in]
          n677 = call "Read connection.vi"("error in (no error)"=w1755, "Server in"=w1756) -> ("error out"=w1754:errorcluster, "connection"=w1717:bool)  [unwired: 7 in, 1 out]
          n678 = case shown="False" w1717 {
            tunnel: [u8 6 ("TRIGGER_MODE") u8 0 ("TRIGGER_MODE")] -> w1716
            frame True {
            }
            frame False {
            }
          }
          n679 = call-dynamic "Read AcquisitionD.vi"("error in (no error)"=w1754, "S4ACS_GUI in"=w1751) -> ("error out"=w1738:errorcluster, "Acquisition.lvclass"=w1739:refnum<class "Acquisition.lvclass">, "S4ACS_GUI out"=w1737:refnum<class "S4GUI.lvclass">)  [unwired: 7 in]
          n680 = call-dynamic "Read Channel.vi"("error in (no error)"=w1738, "Acquisition in"=w1739) -> ("error out"=w1722:errorcluster, "Channel.lvclass"=w1721:refnum<class "Channel.lvclass">, "Acquisition out"=w1748:refnum<class "Acquisition.lvclass">)  [unwired: 7 in]
          n681 = call-dynamic "Read Interface.vi"("error in (no error)"=w1722, "Channel in"=w1721) -> ("error out"=w1720:errorcluster, "Interface.lvclass"=w1726:refnum<class "Interface.lvclass">, "Channel out"=w1725:refnum<class "Channel.lvclass">)  [unwired: 7 in]
          n682 = call-dynamic "Get CCD_Config.vi"("error in (no error)"=w1720, "Interface in"=w1726) -> ("error out"=w1733:errorcluster, "output cluster"=w1734:T1, "Interface out"=w1732:refnum<class "Interface.lvclass">)  [unwired: 7 in]
          n683 = Bundle By Name(cluster=w1734, "TRIGGER_MODE"=w1716) -> (w1731:T1)
          n684 = call-dynamic "Set CCD_Config.vi"("error in (no error)"=w1733, "input cluster"=w1731, "Interface in"=w1732) -> ("error out"=w1729:errorcluster, "Interface out"=w1727:refnum<class "Interface.lvclass">)  [unwired: 7 in]
          n685 = Flatten To String(anything=w1731, error in (no error)=w1729) -> (data string=w1730:string, error out=w1728:errorcluster)  [unwired: 2 in, 1 out]
          n686 = call "Write flatted cluster.vi"("error in (no error)"=w1728, "flatted cluster"=w1730, "Interface in"=w1727) -> ("error out"=w1723:errorcluster, "Interface out"=w1724:refnum<class "Interface.lvclass">)  [unwired: 7 in]
          n687 = call-dynamic "Write Interface.vi"("error in (no error)"=w1723, "Interface.lvclass"=w1724, "Channel in"=w1725) -> ("error out"=w1719:errorcluster, "Channel out"=w1718:refnum<class "Channel.lvclass">)  [unwired: 7 in]
          n688 = call-dynamic "Read State Machine.vi"("error in (no error)"=w1719, "Device in"=w1718) -> ("error out"=w1745:errorcluster, "State Machine.lvclass"=w1747:refnum<class "State Machine.lvclass">, "Device out"=w1743:refnum<class "Channel.lvclass">)  [unwired: 7 in]
          n689 = Increment(x=w1759) -> (x+1=w1758:u32)
          n690 = call "Next State.vi"("error in (no error)"=w1745, "New_State"=60, "State Machine in"=w1747) -> ("error out"=w1740:errorcluster, "State Machine out"=w1741:refnum<class "State Machine.lvclass">)  [unwired: 7 in]
          n691 = call-dynamic "Write State Machine.vi"("error in (no error)"=w1740, "State Machine.lvclass"=w1741, "Device in"=w1743) -> ("error out"=w1742:errorcluster, "Device out"=w1744:refnum<class "Channel.lvclass">)  [unwired: 7 in]
          n692 = call-dynamic "Write Channel.vi"("error in (no error)"=w1742, "Channel.lvclass"=w1744, "Acquisition in"=w1748) -> ("error out"=w1735:errorcluster, "Acquisition out"=w1736:refnum<class "Acquisition.lvclass">)  [unwired: 7 in]
          n693 = call-dynamic "Write AcquisitionD.vi"("error in (no error)"=w1735, "Acquisition.lvclass"=w1736, "S4ACS_GUI in"=w1737) -> ("error out"=w1750:errorcluster, "S4ACS_GUI out"=w1749:refnum<class "S4GUI.lvclass">)  [unwired: 7 in]
          n694 = Bundle By Name(cluster=w1749, "Obs_state"=w1758) -> (w1757:refnum<class "S4GUI.lvclass">)
        }
        frame 266 {
          # "Espera terminar a execução do comando atual \nantes de ir ao proximo passo da Observação."
          n695 = call-dynamic "Read AcquisitionD.vi"("error in (no error)"=w1779, "S4ACS_GUI in"=w1780) -> ("error out"=w1785:errorcluster, "Acquisition.lvclass"=w1786:refnum<class "Acquisition.lvclass">, "S4ACS_GUI out"=w1782:refnum<class "S4GUI.lvclass">)  [unwired: 7 in]
          n696 = call-dynamic "Read Channel.vi"("error in (no error)"=w1785, "Acquisition in"=w1786) -> ("error out"=w1777:errorcluster, "Channel.lvclass"=w1776:refnum<class "Channel.lvclass">, "Acquisition out"=w1784:refnum<class "Acquisition.lvclass">)  [unwired: 7 in]
          n697 = call-dynamic "Read State Machine.vi"("error in (no error)"=w1777, "Device in"=w1776) -> ("error out"=w1768:errorcluster, "State Machine.lvclass"=w1770:refnum<class "State Machine.lvclass">, "Device out"=w1774:refnum<class "Channel.lvclass">)  [unwired: 7 in]
          n698 = call-dynamic "Read State.vi"("error in (no error)"=w1768, "State Machine in"=w1770) -> ("error out"=w1767:errorcluster, "State"=w1764:i32, "State Machine out"=w1769:refnum<class "State Machine.lvclass">)  [unwired: 7 in]
          n699 = Equal To 0?(x=w1764) -> (x = 0?=w1766:bool)
          n700 = call-dynamic "Write State Machine.vi"("error in (no error)"=w1767, "State Machine.lvclass"=w1769, "Device in"=w1774) -> ("error out"=w1773:errorcluster, "Device out"=w1775:refnum<class "Channel.lvclass">)  [unwired: 7 in]
          n701 = call-dynamic "Write Channel.vi"("error in (no error)"=w1773, "Channel.lvclass"=w1775, "Acquisition in"=w1784) -> ("error out"=w1781:errorcluster, "Acquisition out"=w1783:refnum<class "Acquisition.lvclass">)  [unwired: 7 in]
          n702 = Select(t=u32 299, s=w1766, f=w1763) -> (s? t:f=w1765:u32)
          n703 = call-dynamic "Write AcquisitionD.vi"("error in (no error)"=w1781, "Acquisition.lvclass"=w1783, "S4ACS_GUI in"=w1782) -> ("error out"=w1778:errorcluster, "S4ACS_GUI out"=w1772:refnum<class "S4GUI.lvclass">)  [unwired: 7 in]
          n704 = Bundle By Name(cluster=w1772, "Obs_state"=w1765) -> (w1771:refnum<class "S4GUI.lvclass">)
        }
        frame 271 {
          # "Prepara os canais de aquisição para sequencia de foco...."
          n705 = flat-sequence {
            tunnel: w1813 -> [w1918]
            tunnel: [w1918] -> w1812
            frame #0 {
              n706 = Tick Count (ms)() -> (millisecond timer value=→"time5":u32)
            }
          }
          n707 = call-dynamic "Read AcquisitionA.vi"("error in (no error)"=w1812, "S4ACS_GUI in"=w1834) -> ("error out"=w1832:errorcluster, "Acquisition.lvclass"=w1833:refnum<class "Acquisition.lvclass">, "S4ACS_GUI out"=w1836:refnum<class "S4GUI.lvclass">)  [unwired: 7 in]
          n708 = call "Read connection.vi"("error in (no error)"=w1832, "Server in"=w1833) -> ("error out"=w1831:errorcluster, "connection"=w1811:bool, "Server out"=w1830:refnum<class "Acquisition.lvclass">)  [unwired: 7 in]
          n709 = case shown="True" w1811 {
            tunnel: [w1899 w1917] -> w1837
            tunnel: [w1898 w1916] -> w1835
            tunnel: w1831 -> [w1898 w1915]
            tunnel: w1830 -> [w1899 w1914]
            frame False {
            }
            frame True {
              # "configura o canal,\nmas não dispara\na exposicao."
              n710 = call-dynamic "Read Channel.vi"("error in (no error)"=w1915, "Acquisition in"=w1914) -> ("error out"=w1904:errorcluster, "Channel.lvclass"=w1906:refnum<class "Channel.lvclass">, "Acquisition out"=w1913:refnum<class "Acquisition.lvclass">)  [unwired: 7 in]
              n711 = call-dynamic "Write expose.vi"("error in (no error)"=w1904, "expose"=FALSE, "Channel in"=w1906) -> ("error out"=w1903:errorcluster, "Channel out"=w1905:refnum<class "Channel.lvclass">)  [unwired: 7 in]
              n712 = call-dynamic "Read State Machine.vi"("error in (no error)"=w1903, "Device in"=w1905) -> ("error out"=w1910:errorcluster, "State Machine.lvclass"=w1912:refnum<class "State Machine.lvclass">, "Device out"=w1908:refnum<class "Channel.lvclass">)  [unwired: 7 in]
              n713 = call "Next State.vi"("error in (no error)"=w1910, "New_State"=1, "State Machine in"=w1912) -> ("error out"=w1900:errorcluster, "State Machine out"=w1901:refnum<class "State Machine.lvclass">)  [unwired: 7 in]
              n714 = call-dynamic "Write State Machine.vi"("error in (no error)"=w1900, "State Machine.lvclass"=w1901, "Device in"=w1908) -> ("error out"=w1907:errorcluster, "Device out"=w1909:refnum<class "Channel.lvclass">)  [unwired: 7 in]
              n715 = call-dynamic "Write Channel.vi"("error in (no error)"=w1907, "Channel.lvclass"=w1909, "Acquisition in"=w1913) -> ("error out"=w1916:errorcluster, "Acquisition out"=w1917:refnum<class "Acquisition.lvclass">)  [unwired: 7 in]
            }
          }
          n716 = Increment(x=w1829) -> (x+1=w1793:u32)
          n717 = call-dynamic "Write AcquisitionA.vi"("error in (no error)"=w1835, "Acquisition.lvclass"=w1837, "S4ACS_GUI in"=w1836) -> ("error out"=w1825:errorcluster, "S4ACS_GUI out"=w1824:refnum<class "S4GUI.lvclass">)  [unwired: 7 in]
          n718 = call "Read AcquisitionB.vi"("error in (no error)"=w1825, "S4ACS_GUI in"=w1824) -> ("error out"=w1826:errorcluster, "Acquisition.lvclass"=w1827:refnum<class "Acquisition.lvclass">, "S4ACS_GUI out"=w1828:refnum<class "S4GUI.lvclass">)  [unwired: 7 in]
          n719 = call "Read connection.vi"("error in (no error)"=w1826, "Server in"=w1827) -> ("error out"=w1809:errorcluster, "connection"=w1808:bool, "Server out"=w1810:refnum<class "Acquisition.lvclass">)  [unwired: 7 in]
          n720 = case shown="True" w1808 {
            tunnel: [w1879 w1897] -> w1807
            tunnel: [w1878 w1896] -> w1806
            tunnel: w1809 -> [w1878 w1895]
            tunnel: w1810 -> [w1879 w1894]
            frame False {
            }
            frame True {
              # "configura o canal,\nmas não dispara\na exposicao."
              n721 = call-dynamic "Read Channel.vi"("error in (no error)"=w1895, "Acquisition in"=w1894) -> ("error out"=w1884:errorcluster, "Channel.lvclass"=w1886:refnum<class "Channel.lvclass">, "Acquisition out"=w1893:refnum<class "Acquisition.lvclass">)  [unwired: 7 in]
              n722 = call-dynamic "Write expose.vi"("error in (no error)"=w1884, "expose"=FALSE, "Channel in"=w1886) -> ("error out"=w1883:errorcluster, "Channel out"=w1885:refnum<class "Channel.lvclass">)  [unwired: 7 in]
              n723 = call-dynamic "Read State Machine.vi"("error in (no error)"=w1883, "Device in"=w1885) -> ("error out"=w1890:errorcluster, "State Machine.lvclass"=w1892:refnum<class "State Machine.lvclass">, "Device out"=w1888:refnum<class "Channel.lvclass">)  [unwired: 7 in]
              n724 = call "Next State.vi"("error in (no error)"=w1890, "New_State"=1, "State Machine in"=w1892) -> ("error out"=w1880:errorcluster, "State Machine out"=w1881:refnum<class "State Machine.lvclass">)  [unwired: 7 in]
              n725 = call-dynamic "Write State Machine.vi"("error in (no error)"=w1880, "State Machine.lvclass"=w1881, "Device in"=w1888) -> ("error out"=w1887:errorcluster, "Device out"=w1889:refnum<class "Channel.lvclass">)  [unwired: 7 in]
              n726 = call-dynamic "Write Channel.vi"("error in (no error)"=w1887, "Channel.lvclass"=w1889, "Acquisition in"=w1893) -> ("error out"=w1896:errorcluster, "Acquisition out"=w1897:refnum<class "Acquisition.lvclass">)  [unwired: 7 in]
            }
          }
          n727 = call "Write AcquisitionB.vi"("error in (no error)"=w1806, "Acquisition.lvclass"=w1807, "S4ACS_GUI in"=w1828) -> ("error out"=w1817:errorcluster, "S4ACS_GUI out"=w1816:refnum<class "S4GUI.lvclass">)  [unwired: 7 in]
          n728 = call-dynamic "Read AcquisitionC.vi"("error in (no error)"=w1817, "S4ACS_GUI in"=w1816) -> ("error out"=w1821:errorcluster, "Acquisition.lvclass"=w1822:refnum<class "Acquisition.lvclass">, "S4ACS_GUI out"=w1823:refnum<class "S4GUI.lvclass">)  [unwired: 7 in]
          n729 = call "Read connection.vi"("error in (no error)"=w1821, "Server in"=w1822) -> ("error out"=w1803:errorcluster, "connection"=w1804:bool, "Server out"=w1805:refnum<class "Acquisition.lvclass">)  [unwired: 7 in]
          n730 = case shown="True" w1804 {
            tunnel: [w1859 w1877] -> w1802
            tunnel: [w1858 w1876] -> w1801
            tunnel: w1803 -> [w1858 w1875]
            tunnel: w1805 -> [w1859 w1874]
            frame False {
            }
            frame True {
              # "configura o canal,\nmas não dispara\na exposicao."
              n731 = call-dynamic "Read Channel.vi"("error in (no error)"=w1875, "Acquisition in"=w1874) -> ("error out"=w1864:errorcluster, "Channel.lvclass"=w1866:refnum<class "Channel.lvclass">, "Acquisition out"=w1873:refnum<class "Acquisition.lvclass">)  [unwired: 7 in]
              n732 = call-dynamic "Write expose.vi"("error in (no error)"=w1864, "expose"=FALSE, "Channel in"=w1866) -> ("error out"=w1863:errorcluster, "Channel out"=w1865:refnum<class "Channel.lvclass">)  [unwired: 7 in]
              n733 = call-dynamic "Read State Machine.vi"("error in (no error)"=w1863, "Device in"=w1865) -> ("error out"=w1870:errorcluster, "State Machine.lvclass"=w1872:refnum<class "State Machine.lvclass">, "Device out"=w1868:refnum<class "Channel.lvclass">)  [unwired: 7 in]
              n734 = call "Next State.vi"("error in (no error)"=w1870, "New_State"=1, "State Machine in"=w1872) -> ("error out"=w1860:errorcluster, "State Machine out"=w1861:refnum<class "State Machine.lvclass">)  [unwired: 7 in]
              n735 = call-dynamic "Write State Machine.vi"("error in (no error)"=w1860, "State Machine.lvclass"=w1861, "Device in"=w1868) -> ("error out"=w1867:errorcluster, "Device out"=w1869:refnum<class "Channel.lvclass">)  [unwired: 7 in]
              n736 = call-dynamic "Write Channel.vi"("error in (no error)"=w1867, "Channel.lvclass"=w1869, "Acquisition in"=w1873) -> ("error out"=w1876:errorcluster, "Acquisition out"=w1877:refnum<class "Acquisition.lvclass">)  [unwired: 7 in]
            }
          }
          n737 = call-dynamic "Write AcquisitionC.vi"("error in (no error)"=w1801, "Acquisition.lvclass"=w1802, "S4ACS_GUI in"=w1823) -> ("error out"=w1815:errorcluster, "S4ACS_GUI out"=w1814:refnum<class "S4GUI.lvclass">)  [unwired: 7 in]
          n738 = call-dynamic "Read AcquisitionD.vi"("error in (no error)"=w1815, "S4ACS_GUI in"=w1814) -> ("error out"=w1818:errorcluster, "Acquisition.lvclass"=w1819:refnum<class "Acquisition.lvclass">, "S4ACS_GUI out"=w1820:refnum<class "S4GUI.lvclass">)  [unwired: 7 in]
          n739 = call "Read connection.vi"("error in (no error)"=w1818, "Server in"=w1819) -> ("error out"=w1798:errorcluster, "connection"=w1800:bool, "Server out"=w1799:refnum<class "Acquisition.lvclass">)  [unwired: 7 in]
          n740 = case shown="True" w1800 {
            tunnel: [w1839 w1857] -> w1797
            tunnel: [w1838 w1856] -> w1796
            tunnel: w1798 -> [w1838 w1855]
            tunnel: w1799 -> [w1839 w1854]
            frame False {
            }
            frame True {
              # "configura o canal,\nmas não dispara\na exposicao."
              n741 = call-dynamic "Read Channel.vi"("error in (no error)"=w1855, "Acquisition in"=w1854) -> ("error out"=w1844:errorcluster, "Channel.lvclass"=w1846:refnum<class "Channel.lvclass">, "Acquisition out"=w1853:refnum<class "Acquisition.lvclass">)  [unwired: 7 in]
              n742 = call-dynamic "Write expose.vi"("error in (no error)"=w1844, "expose"=FALSE, "Channel in"=w1846) -> ("error out"=w1843:errorcluster, "Channel out"=w1845:refnum<class "Channel.lvclass">)  [unwired: 7 in]
              n743 = call-dynamic "Read State Machine.vi"("error in (no error)"=w1843, "Device in"=w1845) -> ("error out"=w1850:errorcluster, "State Machine.lvclass"=w1852:refnum<class "State Machine.lvclass">, "Device out"=w1848:refnum<class "Channel.lvclass">)  [unwired: 7 in]
              n744 = call "Next State.vi"("error in (no error)"=w1850, "New_State"=1, "State Machine in"=w1852) -> ("error out"=w1840:errorcluster, "State Machine out"=w1841:refnum<class "State Machine.lvclass">)  [unwired: 7 in]
              n745 = call-dynamic "Write State Machine.vi"("error in (no error)"=w1840, "State Machine.lvclass"=w1841, "Device in"=w1848) -> ("error out"=w1847:errorcluster, "Device out"=w1849:refnum<class "Channel.lvclass">)  [unwired: 7 in]
              n746 = call-dynamic "Write Channel.vi"("error in (no error)"=w1847, "Channel.lvclass"=w1849, "Acquisition in"=w1853) -> ("error out"=w1856:errorcluster, "Acquisition out"=w1857:refnum<class "Acquisition.lvclass">)  [unwired: 7 in]
            }
          }
          n747 = call-dynamic "Write AcquisitionD.vi"("error in (no error)"=w1796, "Acquisition.lvclass"=w1797, "S4ACS_GUI in"=w1820) -> ("error out"=w1788:errorcluster, "S4ACS_GUI out"=w1792:refnum<class "S4GUI.lvclass">)  [unwired: 7 in]
          n748 = Unbundle By Name(w1792) -> ("TelFocus.lvclass"=w1791:refnum<class "TelFocus.lvclass">)
          n749 = call-dynamic "Write focus #stepsdone.vi"("error in (no error)"=w1788, "focus #stepsdone"=u32 0, "TelFocus in"=w1791) -> ("error out"=w1787:errorcluster, "TelFocus out"=w1789:refnum<class "TelFocus.lvclass">)  [unwired: 7 in]
          n750 = Bundle By Name(cluster=w1792, "TelFocus.lvclass"=w1789, "Error Msg"="", "Obs_state"=w1793) -> (w1794:refnum<class "S4GUI.lvclass">)
        }
        frame 272 {
          w1928 = 38 ("x")
          w1937 = 28 ("x")
          # "Se algum canal foi pra 38: Texp inválido \npara a configuração do CCD."
          # "Se algum canal foi pra 28: ERRO na inicialização."
          # "Espera terminar a execução da preparação\ndos 4 canais antes de ir ao proximo passo \nda Observação."
          n751 = flat-sequence {
            tunnel: w1970 -> [w2075]
            tunnel: [w2075] -> w1969
            frame #0 {
              n752 = Tick Count (ms)() -> (millisecond timer value=→"time6":u32)
            }
          }
          n753 = call-dynamic "Read AcquisitionA.vi"("error in (no error)"=w1969, "S4ACS_GUI in"=w1980) -> ("error out"=w1967:errorcluster, "Acquisition.lvclass"=w1968:refnum<class "Acquisition.lvclass">, "S4ACS_GUI out"=w1982:refnum<class "S4GUI.lvclass">)  [unwired: 7 in]
          n754 = call "Read connection.vi"("error in (no error)"=w1967, "Server in"=w1968) -> ("error out"=w1965:errorcluster, "connection"=w1964:bool, "Server out"=w1966:refnum<class "Acquisition.lvclass">)  [unwired: 7 in]
          n755 = case shown="True" w1964 {
            tunnel: w1966 -> [w2058 w2074]
            tunnel: w1965 -> [w2057 w2073]
            tunnel: [w2058 w2071] -> w1983
            tunnel: [w2057 w2070] -> w1981
            tunnel: [0 ("State") w2060] -> w1927
            frame False {
            }
            frame True {
              n756 = call-dynamic "Read Channel.vi"("error in (no error)"=w2073, "Acquisition in"=w2074) -> ("error out"=w2069:errorcluster, "Channel.lvclass"=w2068:refnum<class "Channel.lvclass">, "Acquisition out"=w2072:refnum<class "Acquisition.lvclass">)  [unwired: 7 in]
              n757 = call-dynamic "Read State Machine.vi"("error in (no error)"=w2069, "Device in"=w2068) -> ("error out"=w2062:errorcluster, "State Machine.lvclass"=w2064:refnum<class "State Machine.lvclass">, "Device out"=w2066:refnum<class "Channel.lvclass">)  [unwired: 7 in]
              n758 = call-dynamic "Read State.vi"("error in (no error)"=w2062, "State Machine in"=w2064) -> ("error out"=w2061:errorcluster, "State"=w2060:i32, "State Machine out"=w2063:refnum<class "State Machine.lvclass">)  [unwired: 7 in]
              n759 = call-dynamic "Write State Machine.vi"("error in (no error)"=w2061, "State Machine.lvclass"=w2063, "Device in"=w2066) -> ("error out"=w2065:errorcluster, "Device out"=w2067:refnum<class "Channel.lvclass">)  [unwired: 7 in]
              n760 = call-dynamic "Write Channel.vi"("error in (no error)"=w2065, "Channel.lvclass"=w2067, "Acquisition in"=w2072) -> ("error out"=w2070:errorcluster, "Acquisition out"=w2071:refnum<class "Acquisition.lvclass">)  [unwired: 7 in]
            }
          }
          n761 = call-dynamic "Write AcquisitionA.vi"("error in (no error)"=w1981, "Acquisition.lvclass"=w1983, "S4ACS_GUI in"=w1982) -> ("error out"=w1977:errorcluster, "S4ACS_GUI out"=w1976:refnum<class "S4GUI.lvclass">)  [unwired: 7 in]
